vi "WindSpeedInput.vi"(6 "Elapsed Time Reset Control (s)":dbl=20.0 format="%#_13g") -> (10 "?":bool, 14 "Wind Speed":dbl, 16 "Wind Frequency (Hz)":dbl, 17 "Time between previous two clicks (s)":dbl, 19 "Time elapsed after a click (s)":dbl caption="Elapsed Time (s)")   [LabVIEW 2016]
doc: "This VI calculates the wind speed from the anemometer signal. \nInputs: Reset control for time elapsed (to reset wind speed to zero)\nOutputs: Digital Signal from anemometer, Wind speed (MPH), Wind frequency (Hz), time between two clicks of the anemometer (s), time elapsed after a click (s), Anemometer clicks"
uses:
  <vilib>/myRIO/Instrument Drivers/Onboard IO/DIO/typedefs/DIO Reference.ctl
  <vilib>/myRIO/Common/Instrument Driver Framework/Utilities/typedefs/myRIO Generic Hardware Reference.ctl
  <vilib>/myRIO/Common/Instrument Driver Framework/Utilities/typedefs/Hardware Version Enum.ctl
  <vilib>/myRIO/Common/Instrument Driver Framework/Utilities/typedefs/myRIO v1.0 Reference.ctl
  <vilib>/myRIO/Common/Instrument Driver Framework/Utilities/typedefs/Generic FPGA Reference.ctl
  <vilib>/myRIO/Common/Instrument Driver Framework/myRIO v1.0/DIO/typedefs/DIO Channels List.ctl
  <vilib>/myRIO/Common/Instrument Driver Framework/myRIO v1.0/DIO/typedefs/DIO Channels Enum.ctl
  <vilib>/userdefined/High Color/nirio_resource_hc.ctl
  <vilib>/myRIO/Common/Instrument Driver Framework/Utilities/vis/Is FPGA Ref Available.vi
  <vilib>/myRIO/Common/Instrument Driver Framework/myRIO v1.0/DIO/vis/myRIO v1.1 Open DIO.vi
  <vilib>/myRIO/Instrument Drivers/Onboard IO/DIO/vis/Read.vi
  <vilib>/myRIO/Common/Instrument Driver Framework/Utilities/vis/Validate Channels.vi
  <vilib>/myRIO/Common/Instrument Driver Framework/myRIO v1.0/DIO/vis/myRIO v1.0 Reserve DIO.vi
  <vilib>/myRIO/Common/Instrument Driver Framework/myRIO v1.0/Resource Manager/vis/myRIO v1.0 Reserve Channel List.vi
  <vilib>/myRIO/Common/Instrument Driver Framework/myRIO v1.0/DIO/vis/myRIO v1.0 Build MUX Configuration DIO.vi
  <vilib>/myRIO/Common/Instrument Driver Framework/myRIO v1.0/Resource Manager/vis/myRIO v1.0 Reserve Channel.vi
  <vilib>/myRIO/Common/Instrument Driver Framework/myRIO v1.0/Resource Manager/vis/myRIO v1.0 Unreserve Channel.vi
  <vilib>/myRIO/Common/Instrument Driver Framework/myRIO v1.0/Resource Manager/vis/myRIO v1.0 Create Configuration List.vi
  <vilib>/myRIO/Common/Instrument Driver Framework/myRIO v1.0/Resource Manager/vis/myRIO v1.0 Build Mutex Name.vi
  <vilib>/Utility/VariantDataType/GetNumericInfo.vi
  <vilib>/Utility/error.llb/Error Cluster From Error Code.vi
  <vilib>/myRIO/Common/Instrument Driver Framework/myRIO v1.0/myRIO v1.1 Open.vi
  <vilib>/myRIO/Common/Instrument Driver Framework/Utilities/vis/IO Manager.vi
  <vilib>/myRIO/Common/Instrument Driver Framework/Utilities/vis/Configuration Manager.vi
  <vilib>/myRIO/Common/Instrument Driver Framework/myRIO v1.0/Resource Manager/vis/myRIO v1.0 Configure IO.vi
  <vilib>/myRIO/Common/Instrument Driver Framework/myRIO v1.0/myRIO v1.0 Close.vi
  <vilib>/myRIO/Common/Instrument Driver Framework/myRIO v1.0/DIO/vis/myRIO v1.0 Read DIO.vi
  <vilib>/myRIO/Express VI/Onboard IO/DI/DI Express VI.xnode
  <vilib>/myRIO/Instrument Drivers/Onboard IO/DIO/vis/myRIO DIO Open.xnode
  <vilib>/myRIO/Instrument Drivers/Onboard IO/DIO/DIO.lvlib
panel:
  out "Number of clicks received":dbl
  out "?":string
  in  "Wind Speed Display Unit":u16(ring) items=["mph display", "kph display"]
  out "?":i16(graph)
  in  "STOP":bool
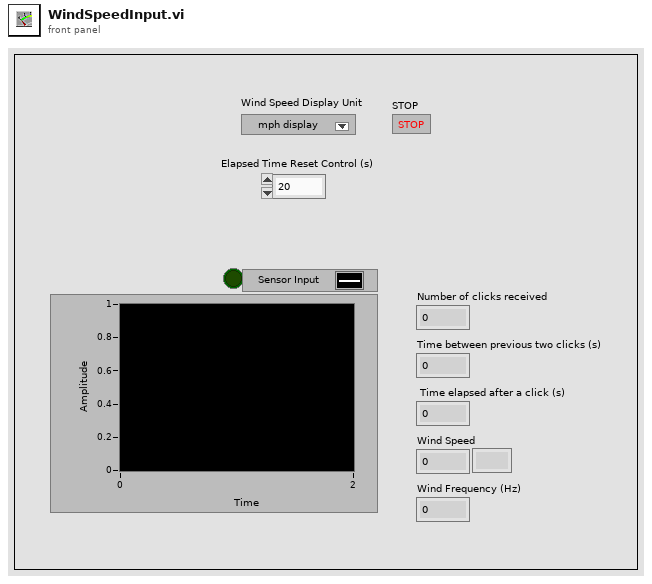
[diagram p1: front panel]
types:
  T1 = typedef "DIO.lvlib/DIO Reference.ctl" = cluster{"myRIO Reference":T2, "DIO Channels List":T6}
  T2 = typedef "myRIO Generic Hardware Reference.ctl" = cluster{"myRIO Model":T3, "myRIO Hardware Reference":T4}
  T3 = typedef "Hardware Version Enum.ctl" = enum16{"Unknown", "myRIO-1900", "myRIO-1950", "roboRIO", "NI ELVIS RIO CM"}
  T4 = typedef "myRIO v1.0 Reference.ctl" = cluster{"Generic FPGA Reference":T5, "Allow multiple opens":bool}
  T5 = typedef "Generic FPGA Reference.ctl" = refnum<k20>
  T6 = typedef "DIO Channels List.ctl" = T7[]
  T7 = typedef "DIO Channels Enum.ctl" = enum16{"Not Connected", "C/DIO0", "C/DIO1", "C/DIO2", "C/DIO3", "C/DIO4", "C/DIO5", "C/DIO6", "C/DIO7", "A/DIO0", "A/DIO1", "A/DIO2", "A/DIO3", "A/DIO4", "A/DIO5", "A/DIO6", "A/DIO7", "A/DIO8", "A/DIO9", "A/DIO10", "A/DIO11", "A/DIO12", "A/DIO13", "A/DIO14", "A/DIO15", "B/DIO0", "B/DIO1", "B/DIO2", "B/DIO3", "B/DIO4", "B/DIO5", "B/DIO6", "B/DIO7", "B/DIO8", "B/DIO9", "B/DIO10", "B/DIO11", "B/DIO12", "B/DIO13", "B/DIO14", "B/DIO15", "LED0", "LED1", "LED2", "LED3", "Button0", "DIO/DIO0", "DIO/DIO1", "DIO/DIO2", "DIO/DIO3", "DIO/DIO4", "DIO/DIO5", "DIO/DIO6", "DIO/DIO7", "DIO/DIO8", "DIO/DIO9", "SPI/CS0", "SPI/CS1", "SPI/CS2", "SPI/CS3", "LED RADIO (Green)", "LED RADIO (Red)", "LED COMM (Green)", "LED COMM (Red)", "LED MODE (Green)", "LED MODE (Red)"}
  T8 = typedef "nirio_resource_hc.ctl" = tag
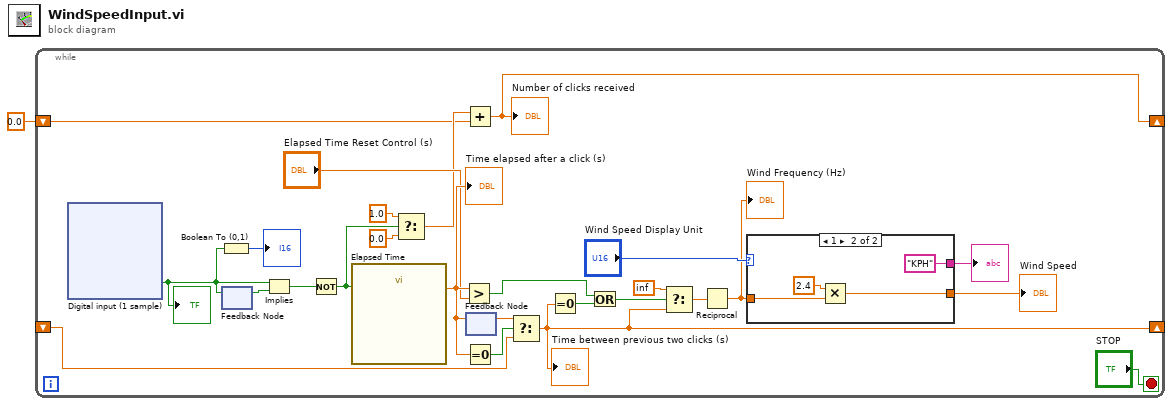
[diagram p0: block diagram]
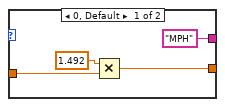
[diagram p2: hidden frame]
diagram:
  n1 = while {
    shift-right: [w14] -> _
    shift-left: _ -> [w15]
    shift-right: [w3] -> _
    shift-left: 0.0 -> [w2]
    stop <- "STOP" stop-if-true
    n2 = xnode "Digital input (1 sample)"() -> ("A/DIO0 (Pin 11)"=w13:bool)  [unwired: 1 in, 1 out]
    "?" <- w13
    n3 = Boolean To (0,1)(Boolean=w13) -> (0, 1=→"?":i16)
    n4 = feedback #1() -> (w17:bool)  [unwired: 1 in]
    n5 = feedback-in #1(w13) -> ()
    n6 = Implies(1:w17, 2:w13) -> (0:w18:bool)
    n7 = Not(x=w18) -> (.not. x?=w7:bool)
    n8 = call "Elapsed Time"("Reset"=w7) -> ("Elapsed Time (s)"=w27:dbl)  [unwired: 11 in, 7 out]
    "Time elapsed after a click (s)" <- w27
    n9 = Select(t=1.0, s=w7, f=0.0) -> (s? t:f=w4:dbl)
    n10 = Greater?(x=w27, y="Elapsed Time Reset Control (s)") -> (0:w24:bool)
    n11 = Add(x=w4, y=w2) -> (x+y=w3:dbl)
    "Number of clicks received" <- w3
    n12 = Equal To 0?(x=w27) -> (x = 0?=w20:bool)
    n13 = feedback #2() -> (w19:dbl)  [unwired: 1 in]
    n14 = feedback-in #2(w27) -> ()
    n15 = Select(t=w19, s=w20, f=w15) -> (s? t:f=w14:dbl)
    "Time between previous two clicks (s)" <- w14
    n16 = Equal To 0?(x=w14) -> (x = 0?=w25:bool)
    n17 = Or(x=w24, y=w25) -> (x .or. y?=w26:bool)
    n18 = Select(t=inf, s=w26, f=w14) -> (s? t:f=w22:dbl)
    n19 = Reciprocal(x=w22) -> (1/x=w10:dbl)
    "Wind Frequency (Hz)" <- w10
    n20 = case shown="1" "Wind Speed Display Unit" {
      tunnel: w10 -> [w31 w34]
      tunnel: [w29 w33] -> w9
      tunnel: ["MPH" ("Unit Label.Text") "KPH" ("Unit Label.Text")] -> w8
      frame 0, Default {
        n21 = Multiply(x=1.492, y=w31) -> (x*y=w29:dbl)
      }
      frame 1 {
        n22 = Multiply(x=2.4, y=w34) -> (x*y=w33:dbl)
      }
    }
    "Wind Speed" <- w9
    "?" <- w8
  }
